vi "Error Handler.vi"(8 "error in":errorcluster, 11 "plugin thread in":refnum<class "Plugin Thread.lvclass">) -> (0 "error out":errorcluster, 3 "plugin thread out":refnum<class "Plugin Thread.lvclass">)   [LabVIEW 2020, in "DSF Core.lvlib" / "Plugin Thread.lvclass"]
uses:
  Thread/Plugin/Plugin Thread.lvclass
  Thread/Thread.lvclass
  C:/Users/nitest/Desktop/Git/niveristand-data-sharing-framework-custom-device/Source/Core/Classes/Thread/Thread.lvclass
  C:/Users/nitest/Desktop/Git/niveristand-data-sharing-framework-custom-device/Source/Core/Classes/Thread/Plugin/Plugin Thread.lvclass
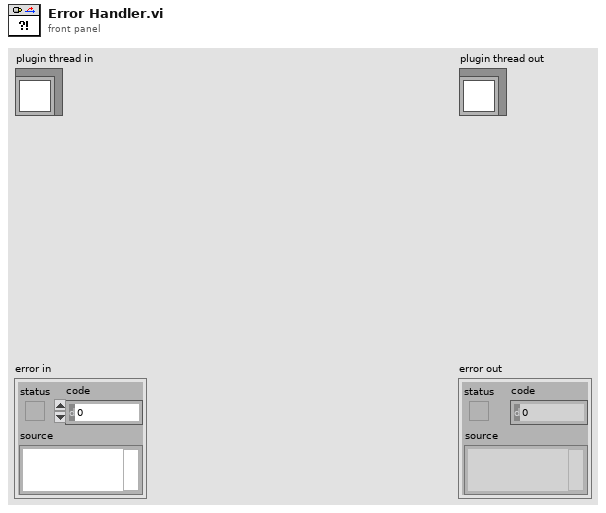
[diagram p1: front panel]
types:
  T1 = typedef "DSF Core.lvlib/Plugin Interface.lvclass/Command.ctl" = enum8{"Idle", "Start", "Set Inline Buffer", "Rx", "Tx", "Shutdown", "Error"}
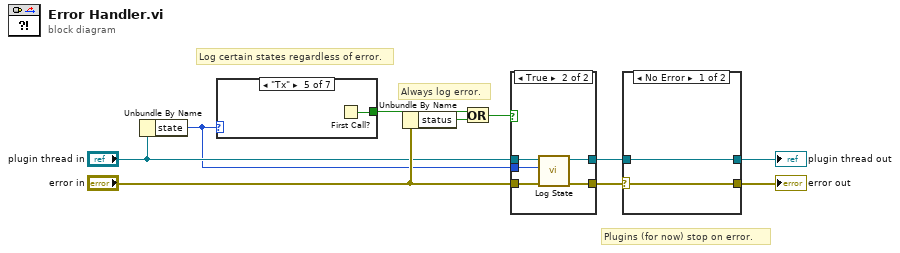
[diagram p0: block diagram]
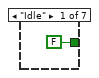
[diagram p2: hidden frame]
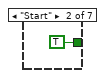
[diagram p3: hidden frame]
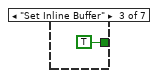
[diagram p4: hidden frame]
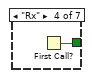
[diagram p5: hidden frame]
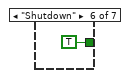
[diagram p6: hidden frame]
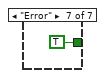
[diagram p7: hidden frame]
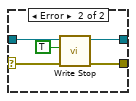
[diagram p9: hidden frame]
diagram:
  # "Plugins (for now) stop on error."
  # "Log certain states regardless of error."
  # "Always log error."
  n1 = Unbundle By Name("plugin thread in") -> ("state"=w1:T1)
  n2 = case shown="\"Tx\"" w1 {
    tunnel: [FALSE ("First Call?: T/F") TRUE TRUE ("status") w14 w15 TRUE ("First Call?: T/F") TRUE ("First Call?: T/F")] -> w10
    frame "Idle" {
    }
    frame "Start" {
    }
    frame "Set Inline Buffer" {
    }
    frame "Rx" {
      n3 = First Call?() -> (First Call?: T/F=w14:bool)
    }
    frame "Tx" {
      n4 = First Call?() -> (First Call?: T/F=w15:bool)
    }
    frame "Shutdown" {
    }
    frame "Error" {
    }
  }
  n5 = Unbundle By Name("error in") -> ("status"=w9:bool)
  n6 = Or(x=w10, y=w9) -> (x .or. y?=w8:bool)
  n7 = case shown="True" w8 {
    tunnel: [w19 w21] -> w5
    tunnel: [w18 w20] -> w6
    tunnel: "plugin thread in" -> [w19 w24]
    tunnel: "error in" -> [w18 w23]
    tunnel: w1 -> [_ w22]
    frame False {
    }
    frame True {
      n8 = call "Log State.vi"("error in (no error)"=w23, "state"=w22, "Plugin Thread in"=w24) -> ("error out"=w20:errorcluster, "Plugin Thread out"=w21:refnum<class "Plugin Thread.lvclass">)  [unwired: 7 in]
    }
  }
  n9 = case shown="No Error" w6 {
    selector: w6 -> [w26 w30]
    tunnel: w5 -> [w25 w29]
    tunnel: [w26 w27] -> w4
    tunnel: [w25 w28] -> w3
    frame No Error {
    }
    frame Error {
      n10 = call "Write Stop.vi"("error in (no error)"=w30, "stop"=TRUE, "Thread in"=w29) -> ("error out"=w27:errorcluster, "Thread out"=w28:refnum<class "Plugin Thread.lvclass">)  [unwired: 7 in]
    }
  }
  "error out" <- w4
  "plugin thread out" <- w3
